vi "MICSD Set 2.45 GHz TX Power.vi"(8 "error in (no error)":errorcluster, 10 "245TX_Power":i8(ring)=10 items=["-29"=-29, "-4"=-4, "-2"=-2, "0"=0, "2"=2, "4"=4, "6"=6, "8"=8, "10"=10, "12"=12, "14"=14, "16"=16, "18"=18, "20"=20, "22"=22, "24"=24, "26"=26, "27"=27], 11 "VISA Resource Name":refnum<visa-resource-name>) -> (0 "error out":errorcluster, 2 "dup 245TX_Power":i8, 3 "dup VISA Resource Name":refnum<visa-resource-name>)   [LabVIEW 2020]
uses:
  <vilib>/Instr/_visa.llb/VISA Configure Serial Port (Instr).vi
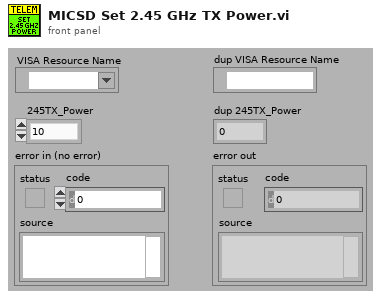
[diagram p1: front panel]
types:
  T1 = cluster{"Command Token":u8, "Length":u16, "Pack Data":u8[]}
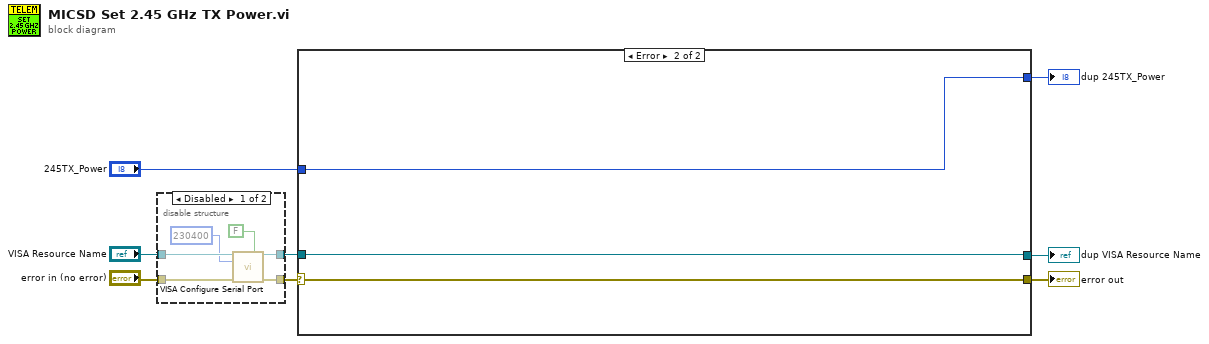
[diagram p0: block diagram]
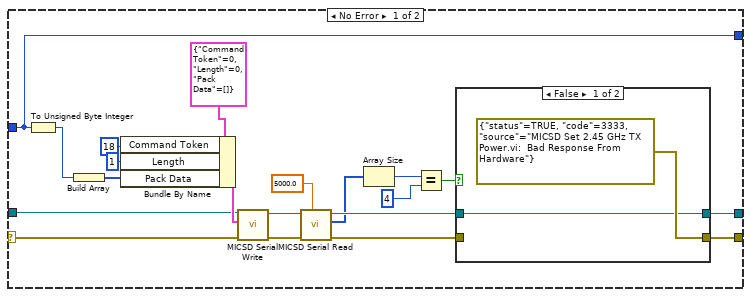
[diagram p3: hidden frame]
diagram:
  n1 = disable-structure shown="Disabled" {
    disable-tunnel: [w14 w15] -> w8
    disable-tunnel: [w13 w16] -> w7
    disable-tunnel: "VISA Resource Name" -> [w12 w16]
    disable-tunnel: "error in (no error)" -> [w11 w15]
    frame Disabled {
      n2 = call-poly "VISA Configure Serial Port"("VISA resource name"=w12, "Enable Termination\nChar (T)"=FALSE ("Enable Termination\nChar (T)"), "baud rate (9600)"=u32 230400, "error in (no error)"=w11) -> ("VISA resource name out"=w13:refnum<visa-resource-name>, "error out"=w14:errorcluster)  [unwired: 10 in]
    }
    frame Enabled {
    }
  }
  n3 = case shown="Error" w8 {
    selector: w8 -> [w28 w43]
    tunnel: [w22 w43] -> w3
    tunnel: w7 -> [w29 w42]
    tunnel: [w24 w42] -> w4
    tunnel: "245TX_Power" -> [w17 w41]
    tunnel: [w17 w41] -> w1
    frame No Error {
      n4 = To Unsigned Byte Integer(number=w17) -> (unsigned 8bit integer=w19:u8)
      n5 = Build Array(w19) -> (w27:u8[])
      n6 = Bundle By Name(cluster=T1 {"Command Token"=0, "Length"=0, "Pack Data"=[]} ("Write Data"), "Command Token"=u8 18, "Length"=u16 1, "Pack Data"=w27) -> (w36:T1)
      n7 = call "MICSD Serial Write.vi"("error in (no error)"=w28, "Write Data"=w36, "VISA Resource Name"=w29) -> ("error out"=w31:errorcluster, "DUP Visa Resource Name"=w34:refnum<visa-resource-name>)  [unwired: 7 in]
      n8 = call "MICSD Serial Read.vi"("Timeout(mS)"=5000.0, "error in (no error)"=w31, "VISA Resource Name"=w34) -> ("error out"=w23:errorcluster, "Read Data"=w18:u8[], "DUP Visa Resource Name"=w25:refnum<visa-resource-name>)  [unwired: 6 in]
      n9 = Array Size(array=w18) -> (size(s)=w21:i32)
      n10 = Equal?(x=w21, y=4) -> (x = y?=w26:bool)
      n11 = case shown="False" w26 {
        tunnel: w25 -> [w37 w40]
        tunnel: [w37 w40] -> w24
        tunnel: w23 -> [_ w39]
        tunnel: [errorcluster {"status"=TRUE, "code"=3333, "source"="MICSD Set 2.45 GHz TX Power.vi:  Bad Response From Hardware"} ("error IO") w39] -> w22
        frame False {
        }
        frame True {
        }
      }
    }
    frame Error {
    }
  }
  "dup VISA Resource Name" <- w4
  "error out" <- w3
  "dup 245TX_Power" <- w1
